vi "PH_Beckhoff.set ADS Error.vi"(0 "i ref in":refnum<vi>, 2 "ADS Error":i32, 5 "error in":errorcluster) -> (14 "i ref out":refnum<vi>, 19 "error out":errorcluster)   [LabVIEW 2014, in "PH_Beckhoff.lvlib"]
doc: "This VI sets the ADS Error to the related GUI element."
uses:
  PH_Beckhoff.lvlib
  non_GPL/instr.lib/Beckhoff/Beckhoff - Driver np.lvlib
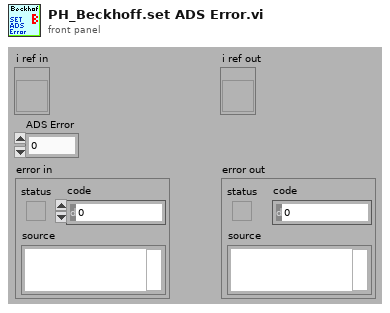
[diagram p1: front panel]
types:
  T1 = typedef "PH_Beckhoff.lvlib/PH_Beckhoff.i attribute.ctl" = cluster{"GUI Refs":T2, "operation?":bool, "Default Prdc Interval":i32, "Connection":T3, "AMS Net ID":T4, "Klemmencluster: # of":T5, "Values":T6, "IP":string, "Description":string, "configured?":bool, "Change Manager":cluster{"Detemination wanted?":bool, "Values changed at":cluster{"Sonderklemmen Inputs":i32[], "Analog Inputs":i32[], "Analog Outputs":i32[], "Digital Inputs":i32[], "Digital Outputs":i32[]}}, "Difference to handle an analog input as change":u32}
  T2 = typedef "PH_Beckhoff.lvlib/PH_Beckhoff.GUI Refs.ctl" = cluster{"ADS Error":refnum<vi>, "Values":refnum<vi>, "configured?":refnum<vi>, "Connection":refnum<vi>, "IP":refnum<vi>, "Prdc Int [ms]":refnum<vi>}
  T3 = typedef "PH_Beckhoff.lvlib/PH_Beckhoff.Connectivity.ctl" = cluster{"DLL?":bool, "Port?":bool, "Client?":bool, "Ping?":bool, "unsuccessful Pings":u32}
  T4 = typedef "Beckhoff - Driver np.lvlib/Beckhoff Access.ctl" = cluster{"DLL path":path, "AMS Net ID":cluster{"1st # of IP":u8, "2nd # of IP":u8, "3rd # of IP":u8, "4th # of IP":u8, "In Port":u8, "Out Port":u8}}
  T5 = typedef "Beckhoff - Driver np.lvlib/Klemmendeclarer.ctl" = cluster{"Offset due to Sonderklemms":u32, "analog Inputs":u32, "analog Outputs":u32, "digital Input Bits":u32, "digital Output Bits":u32}
  T6 = typedef "PH_Beckhoff.lvlib/PH_Beckhoff.Values.ctl" = cluster{"Sonderklemmen Inputs":T7, "Analog Inputs":T8, "Analog Outputs":T10, "Digital Inputs":T11, "Digital Outputs":T12}
  T7 = typedef "PH_Beckhoff.lvlib/PH_Beckhoff.Sonderklemmen Inputs.ctl" = cluster{"Total Length":u32, "Name":string, "Value":u64, "Quality":bool, "Service ID":i32, "Offset":u32, "Length":u32}[]
  T8 = typedef "PH_Beckhoff.lvlib/PH_Beckhoff.Analog Inputs.ctl" = cluster{"Name":string, "Value":u32, "Quality":bool, "Service ID":i32, "Sca Type":T9}[]
  T9 = typedef "PH_Beckhoff.lvlib/PH_Beckhoff.Scaling Type.ctl" = enum16{"none", "0 ... 15 Bit -> 0 ... 5", "0 ... 15 Bit -> 0 ... 10", "0 ... 15 Bit -> 0 ... 25", "0 ... 15 Bit -> 4 ... 20", "0 ... 15 Bit -> 0 ... 1", "0 ... 15 Bit -> 0 ... 20000", "0 ... 15 Bit -> 0 ... 24000"}
  T10 = typedef "PH_Beckhoff.lvlib/PH_Beckhoff.Analog Outputs.ctl" = cluster{"Name":string, "Value":u32, "Quality":bool, "Wanted Value":u32, "Service ID":i32, "Sca Type":T9}[]
  T11 = typedef "PH_Beckhoff.lvlib/PH_Beckhoff.Digital Inputs.ctl" = cluster{"Name":string, "Value":bool, "Quality":bool, "Service ID":i32, "inverted?":bool}[]
  T12 = typedef "PH_Beckhoff.lvlib/PH_Beckhoff.Digital Outputs.ctl" = cluster{"Name":string, "Value":bool, "Quality":bool, "Wanted Value":bool, "Service ID":i32, "inverted?":bool}[]
  T13 = cluster{"Latest Error":string, "Error List":string[]}
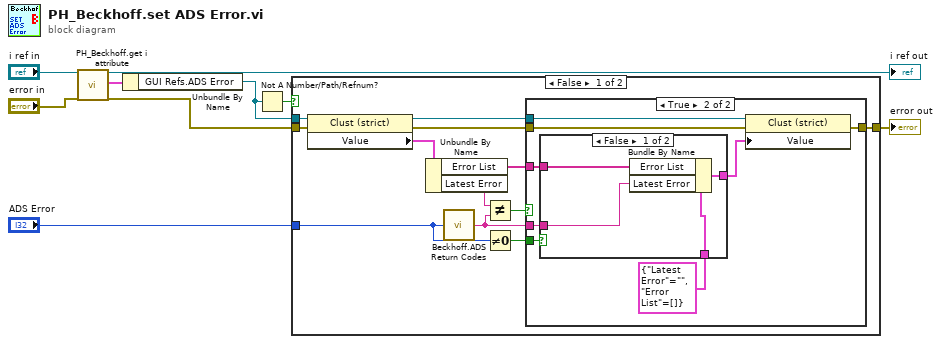
[diagram p0: block diagram]
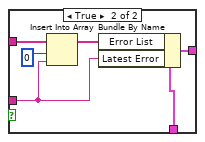
[diagram p3: hidden frame]
diagram:
  n1 = call "PH_Beckhoff.get i attribute.vi"("i ref in"="i ref in", "error in (no error)"="error in") -> ("i ref out"=→"i ref out":refnum<vi>, "i attribute"=w3:T1, "error out"=w6:errorcluster)  [unwired: 15 in]
  n2 = Unbundle By Name(w3) -> ("GUI Refs.ADS Error"=w2:refnum<vi>)
  n3 = Not A Number/Path/Refnum?(number/path/refnum=w2) -> (NaN/Path/Refnum?=w1:bool)
  n4 = case shown="False" w1 {
    tunnel: w6 -> [w21 w41]
    tunnel: [w19 w41] -> w5
    tunnel: "ADS Error" -> [w12 _]
    tunnel: w2 -> [w13 _]
    frame False {
      n5 = property class="Clust (strict)"(reference=w13, error in=w21) -> (reference out=w18:refnum<vi>, error out=w20:errorcluster, "Value"=w17:T13)
      n6 = Unbundle By Name(w17) -> ("Error List"=w15:string[], "Latest Error"=w16:string)
      n7 = call "Beckhoff.ADS Return Codes.vi"("ADS Error"=w12) -> ("Error Code"=w14:string)
      n8 = Not Equal?(x=w16, y=w14) -> (x != y?=w10:bool)
      n9 = Not Equal To 0?(x=w12) -> (x != 0?=w11:bool)
      n10 = case shown="True" w10 {
        tunnel: w20 -> [w22 w30]
        tunnel: [w22 w29] -> w19
        tunnel: w18 -> [_ w28]
        tunnel: w15 -> [_ w27]
        tunnel: w14 -> [_ w25]
        tunnel: w11 -> [_ w24]
        frame False {
        }
        frame True {
          n11 = case shown="False" w24 {
            tunnel: T13 {"Latest Error"="", "Error List"=[]} ("Value") -> [w34 w39]
            tunnel: w27 -> [w31 w38]
            tunnel: [w32 w36] -> w26
            tunnel: w25 -> [w33 w35]
            frame False {
              n12 = Bundle By Name(cluster=w34, "Error List"=w31, "Latest Error"=w33) -> (w32:T13)
            }
            frame True {
              n13 = Insert Into Array(array=w38, index=0, new element=w35) -> (w37:string[])
              n14 = Bundle By Name(cluster=w39, "Error List"=w37, "Latest Error"=w35) -> (w36:T13)
            }
          }
          n15 = property class="Clust (strict)"(reference=w28, error in=w30, "Value"=w26) -> (error out=w29:errorcluster)  [unwired: 1 out]
        }
      }
    }
    frame True {
    }
  }
  "error out" <- w5
